vi "Autonomous Joystick Emulation.vi"() -> ()   [LabVIEW 2011]
panel:
  in  "Crab Joy Angle":dbl
  in  "Crab Joy Magnitude":dbl
  in  "Joy Y Command":dbl
  in  "Joy X Command":dbl
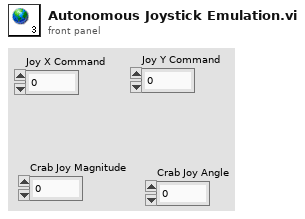
[diagram p1: front panel]
diagram:
